vi "get channels.vi"(8 "error in":errorcluster, 11 "cluster in":variant) -> (0 "error out":errorcluster, 3 "channels":T1[](array[typedef]))   [LabVIEW 2014, in "Scriptable Model Interface Shared.lvlib"]
uses:
  Scriptable Model Interface Shared.lvlib
  <vilib>/Utility/VariantDataType/VariantType.lvlib
  channel id.ctl
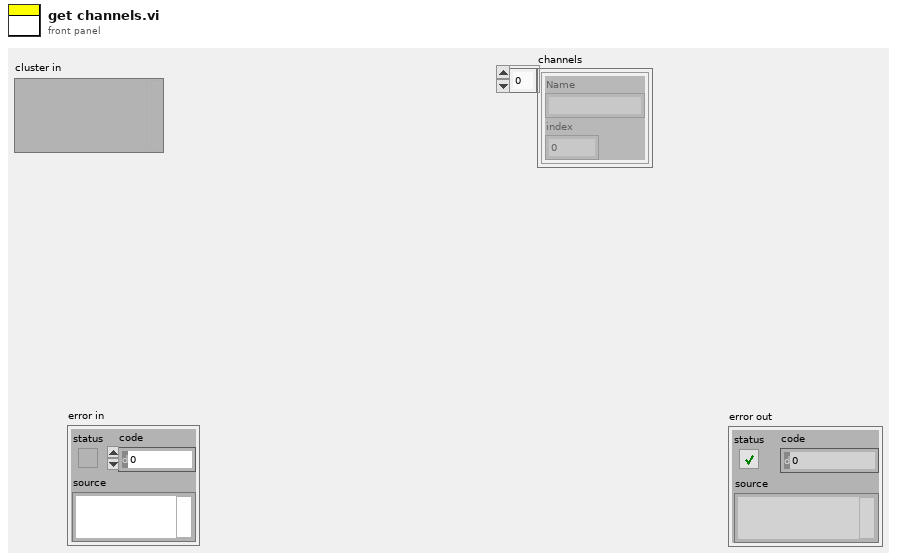
[diagram p1: front panel]
types:
  T1 = typedef "Scriptable Model Interface Shared.lvlib/channel id.ctl" = cluster{"Name":string, "index":i32}
  T2 = typedef "VariantType.lvlib/Type.ctl" = enum8{"Invalid Type", "Void", "I8", "I16", "I32", "I64", "U8", "U16", "U32", "U64", "Single Float", "Double Float", "Extended Float", "Single Complex", "Double Complex", "Extended Complex", "Enum U8", "Enum U16", "Enum U32", "Enum U64", "Single Float With Unit", "Double Float With Unit", "Extended Float With Unit", "Single Complex with Unit", "Double Complex with Unit", "Extended Complex with Unit", "Boolean", "String", "Path", "Picture", "Tag", "Array", "Cluster", "Variant", "LV Variant", "Waveform", "Timestamp", "Digital Waveform", "Digital Data", "ExpressData", "Refnum", "External Data", "VI", "Poly VI", "LabVIEW Class Instance", "Fixed Point"}
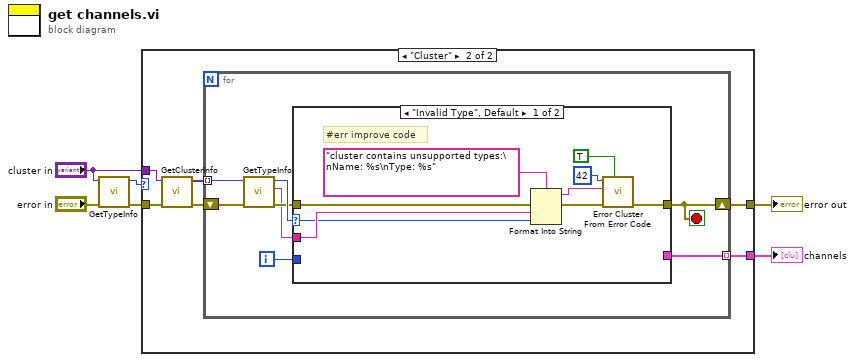
[diagram p0: block diagram]
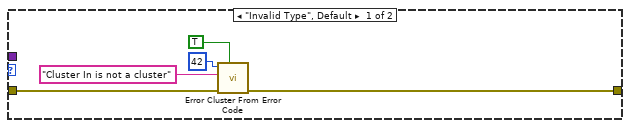
[diagram p2: hidden frame]
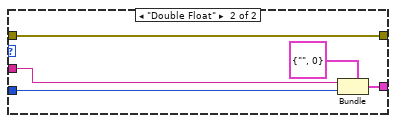
[diagram p3: hidden frame]
diagram:
  n1 = call <vilib>:"GetTypeInfo.vi"("error in (no error)"="error in", "Variant"="cluster in") -> ("error out"=w4:errorcluster, "Type Enum"=w6:T2)  [unwired: 5 in, 3 out]
  n2 = case shown="\"Cluster\"" w6 {
    tunnel: [w11 w13] -> w5
    tunnel: w4 -> [w7 w17]
    tunnel: "cluster in" -> [_ w16]
    tunnel: [_ w12] -> w2
    frame "Invalid Type", Default {
      n3 = call <vilib>:"Error Cluster From Error Code.vi"("show call chain? (False)"=TRUE, "error in (no error)"=w7, "error message (\"\")"="Cluster In is not a cluster" ("error message (\"\")"), "error code (0)"=42) -> ("error out"=w11:errorcluster)  [unwired: 5 in]
    }
    frame "Cluster" {
      n4 = call <vilib>:"GetClusterInfo.vi"("error in (no error)"=w17, "Variant"=w16) -> ("error out"=w14:errorcluster, "Cluster Elements"=w15:variant[])  [unwired: 8 in]
      n5 = for {
        tunnel: w15 -> [w25] mode=indexing
        shift-right: [w21] -> w13
        shift-left: w14 -> [w23]
        tunnel: [w18] -> w12 mode=indexing
        i -> [w19]
        stop <- w21 stop-if-true
        n6 = call <vilib>:"GetTypeInfo.vi"("error in (no error)"=w23, "Variant"=w25) -> ("error out"=w22:errorcluster, "Name"=w20:string, "Type Enum"=w24:T2)  [unwired: 5 in, 2 out]
        n7 = case shown="\"Invalid Type\", Default" w24 {
          selector: w24 -> [w28 _]
          tunnel: [w31 w39] -> w21
          tunnel: w22 -> [w32 w39]
          tunnel: w20 -> [w29 w38]
          tunnel: w19 -> [_ w35]
          tunnel: [_ w37] -> w18
          frame "Invalid Type", Default {
            # "#err improve code"
            n8 = Format Into String(format string="cluster contains unsupported types:\nName: %s\nType: %s" ("error message (\"\")"), error in=w32, w29, w28) -> (resulting string=w26:string, error out=w30:errorcluster)  [unwired: 1 in]
            n9 = call <vilib>:"Error Cluster From Error Code.vi"("show call chain? (False)"=TRUE, "error in (no error)"=w30, "error message (\"\")"=w26, "error code (0)"=42) -> ("error out"=w31:errorcluster)  [unwired: 5 in]
          }
          frame "Double Float" {
            n10 = Bundle(cluster=T1 {"Name"="", "index"=0} ("output cluster"), "Name"=w38, "index"=w35) -> (w37:T1)
          }
        }
      }
    }
  }
  "error out" <- w5
  "channels" <- w2
